vi "Cleanup.vi"(8 "error in (no error)":errorcluster, 11 "Package Builder in":refnum<class "Package Builder.lvclass">) -> (0 "error out":errorcluster, 3 "Package Builder out":refnum<class "Package Builder.lvclass">)   [LabVIEW 2020, in "Package Builder.lvclass"]
uses:
  Package Builder.lvclass
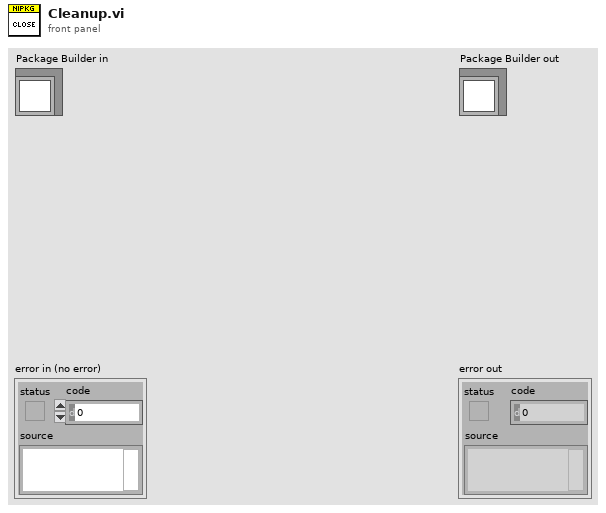
[diagram p1: front panel]
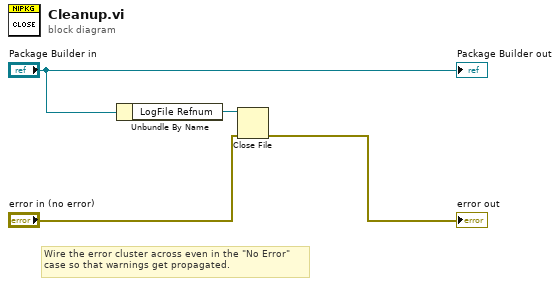
[diagram p0: block diagram]
diagram:
  # "Wire the error cluster across even in the \"No Error\"\ncase so that warnings get propagated."
  n1 = Unbundle By Name("Package Builder in") -> ("LogFile Refnum"=w4:refnum<file>)
  n2 = Close File(refnum=w4, error in="error in (no error)") -> (error out=→"error out":errorcluster)  [unwired: 1 out]
  "Package Builder out" <- "Package Builder in"
